vi "Zero Steer Jaguars.vi"() -> ()   [LabVIEW 2012]
uses:
  Controls/Zero Steer Jags Shifter.ctl
  <vilib>/Rock Robotics/SystemInterfaces/Utilities/FPGA_UtilitiesLED Source.ctl
  <vilib>/Rock Robotics/SystemInterfaces/Utilities/FPGA_UtilitiesLED State.ctl
  <vilib>/Rock Robotics/WPI/Joystick/WPI_JoystickGetSetRefNum.vi
  Globals/Potentiometers.vi
  Globals/Are We Calibrating Steering.vi
  Globals/Jaguar Commands.vi
  Globals/Motor Errors.vi
  Globals/Max Steer Voltage.vi
  <vilib>/Utility/file.llb/Write To Spreadsheet File (DBL).vi
  Globals/Pot Home Values.vi
panel:
  in  "Max Voltage":dbl
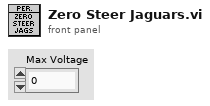
[diagram p1: front panel]
types:
  T1 = typedef "Zero Steer Jags Shifter.ctl" = enum16{"Wait for Button", "Move to Halfway", "Wait for Record"}
  T2 = typedef "WPI_JoystickDevRef.ctl" = cluster{"Device":T3}
  T3 = typedef "WPI_JoystickDeviceEnum.ctl" = enum16{"USB 1", "USB 2", "USB 3", "USB 4", "Kinect 1", "Kinect 2"}
  T4 = typedef "FPGA_UtilitiesLED State.ctl" = enum16{"Off", "On", "Toggle"}
  T5 = typedef "FPGA_UtilitiesLED Source.ctl" = enum16{"User LED", "FPGA LED"}
  T6 = typedef "WPI_AnalogChannelDevRef.ctl" = cluster{"DevStatus":errorcluster, "Analog Module":T7, "Analog Channel":T8}
  T7 = typedef "FPGA_TypedefAnalogModule.ctl" = enum16{"Analog Module 1", "Analog Module 2"}
  T8 = typedef "FPGA_AIChannel.ctl" = enum8{"AI 1", "AI 2", "AI 3", "AI 4", "AI 5", "AI 6", "AI 7", "AI 8", "Invalid"}
  T9 = cluster{"Front Left":T6, "Front Right":T6, "Rear Left":T6, "Rear Right":T6, "Actuator":T6}
  T10 = typedef "WPI_JoystickButtonState.ctl" = cluster{"Button 1":bool, "Button 2":bool, "Button 3":bool, "Button 4":bool, "Button 5":bool, "Button 6":bool, "Button 7":bool, "Button 8":bool, "Button 9":bool, "Button 10":bool, "Button 11":bool, "Button 12":bool}
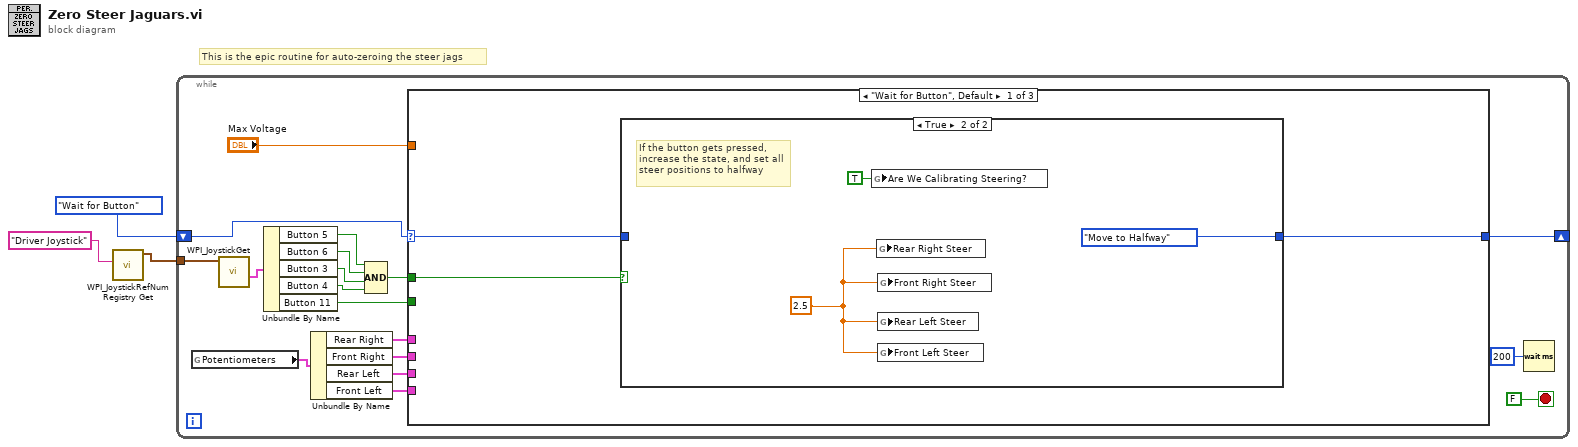
[diagram p0: block diagram]
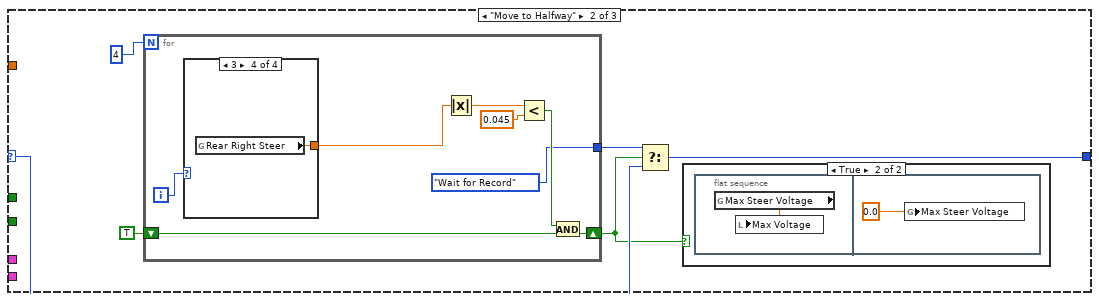
[diagram p3: hidden frame]
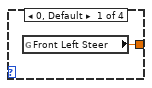
[diagram p5: hidden frame]
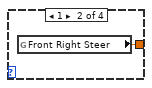
[diagram p6: hidden frame]
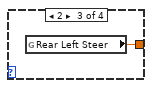
[diagram p7: hidden frame]
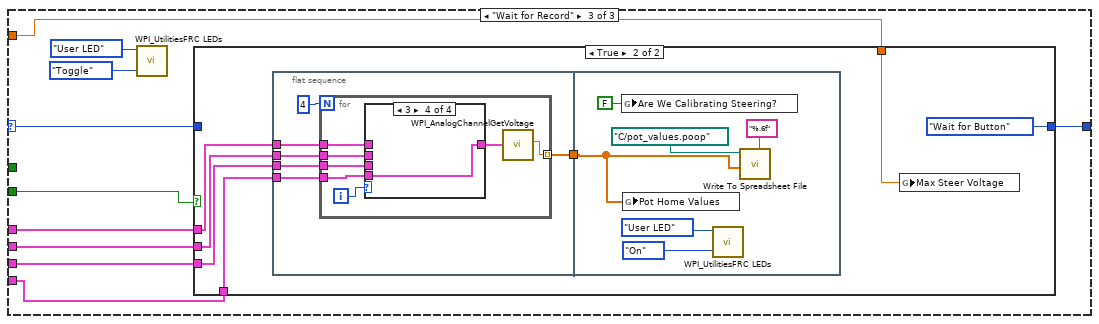
[diagram p8: hidden frame]
diagram:
  # "This is the epic routine for auto-zeroing the steer jags"
  n1 = call <vilib>:"WPI_JoystickRefNum Registry Get.vi"("refnum name"="Driver Joystick") -> ("JoystickDevRef"=w3:T2)  [unwired: 1 in, 9 out]
  n2 = while {
    tunnel: w3 -> [w15]
    shift-right: [w19] -> _
    shift-left: Zero_Steer_Jags_Shifter."Wait for Button" ("States") -> [w20]
    stop <- FALSE stop-if-true
    n3 = global read "Potentiometers.vi" "Potentiometers"() -> (w9:T9)
    n4 = call <vilib>:"WPI_JoystickGet.vi"("JoystickDevRef"=w15) -> ("Buttons"=w17:T10)  [unwired: 4 in, 2 out]
    n5 = Unbundle By Name(w17) -> ("Button 5"=w13:bool, "Button 6"=w12:bool, "Button 3"=w16:bool, "Button 4"=w11:bool, "Button 11"=w10:bool)
    n6 = Unbundle By Name(w9) -> ("Rear Right"=w8:T6, "Front Right"=w7:T6, "Rear Left"=w6:T6, "Front Left"=w5:T6)
    n7 = Compound Arithmetic op=AND(w13, w12, w16, w11) -> (w14:bool)
    n8 = case shown="\"Wait for Button\", Default" w20 {
      selector: w20 -> [w24 w31 w56]
      tunnel: [w23 w32 w55] -> w19
      tunnel: w14 -> [w22 _ _]
      tunnel: w10 -> [_ _ w54]
      tunnel: w8 -> [_ _ w53]
      tunnel: w7 -> [_ _ w52]
      tunnel: w6 -> [_ _ w51]
      tunnel: w5 -> [_ _ w50]
      tunnel: "Max Voltage" -> [_ _ w49]
      frame "Wait for Button", Default {
        n9 = case shown="True" w22 {
          tunnel: w24 -> [w25 _]
          tunnel: [w25 Zero_Steer_Jags_Shifter."Move to Halfway" ("States")] -> w23
          frame False {
          }
          frame True {
            w26 = 2.5 ("Front Right Steer")
            # "If the button gets pressed, \nincrease the state, and set all\nsteer positions to halfway"
            n10 = global write "Are We Calibrating Steering.vi" "Are We Calibrating Steering?"(TRUE ("Are We Calibrating Steering?")) -> ()
            n11 = global write "Jaguar Commands.vi" "Rear Right Steer"(w26) -> ()
            n12 = global write "Jaguar Commands.vi" "Front Right Steer"(w26) -> ()
            n13 = global write "Jaguar Commands.vi" "Rear Left Steer"(w26) -> ()
            n14 = global write "Jaguar Commands.vi" "Front Left Steer"(w26) -> ()
          }
        }
      }
      frame "Move to Halfway" {
        n15 = for {
          N: 4 -> [_]
          shift-right: [w42] -> w29
          shift-left: TRUE -> [w41]
          tunnel: [Zero_Steer_Jags_Shifter."Wait for Record" ("States")] -> w30
          i -> [w44]
          n16 = case shown="3" w44 {
            tunnel: [w45 w46 w47 w48] -> w37
            frame 0, Default {
              n17 = global read "Motor Errors.vi" "Front Left Steer"() -> (w45:dbl)
            }
            frame 1 {
              n18 = global read "Motor Errors.vi" "Front Right Steer"() -> (w46:dbl)
            }
            frame 2 {
              n19 = global read "Motor Errors.vi" "Rear Left Steer"() -> (w47:dbl)
            }
            frame 3 {
              n20 = global read "Motor Errors.vi" "Rear Right Steer"() -> (w48:dbl)
            }
          }
          n21 = Absolute Value(x=w37) -> (abs(x)=w38:dbl)
          n22 = Less?(x=w38, y=0.045) -> (x < y?=w40:bool)
          n23 = And(x=w40, y=w41) -> (x .and. y?=w42:bool)
        }
        n24 = Select(t=w30, s=w29, f=w31) -> (s? t:f=w32:T1)
        n25 = case shown="True" w29 {
          frame False {
          }
          frame True {
            n26 = flat-sequence {
              frame #0 {
                n27 = global read "Max Steer Voltage.vi" "Max Steer Voltage"() -> (w35:dbl)
                n28 = local write "Max Voltage"(w35) -> ()
              }
              frame #1 {
                n29 = global write "Max Steer Voltage.vi" "Max Steer Voltage"(0.0 ("Max Steer Voltage")) -> ()
              }
            }
          }
        }
      }
      frame "Wait for Record" {
        n30 = call <vilib>:"WPI_UtilitiesFRC LEDs.vi"("State"=FPGA_UtilitiesLED_State."Toggle", "LED Type"=FPGA_UtilitiesLED_Source."User LED") -> ()  [unwired: 8 in, 2 out]
        n31 = case shown="True" w54 {
          tunnel: w56 -> [w59 _]
          tunnel: [w59 Zero_Steer_Jags_Shifter."Wait for Button" ("States")] -> w55
          tunnel: w53 -> [_ w65]
          tunnel: w52 -> [_ w64]
          tunnel: w51 -> [_ w63]
          tunnel: w50 -> [_ w62]
          tunnel: w49 -> [_ w60]
          frame False {
          }
          frame True {
            n32 = flat-sequence {
              tunnel: w65 -> [w71]
              tunnel: w64 -> [w70]
              tunnel: w63 -> [w69]
              tunnel: w62 -> [w68]
              tunnel: [w67] -> w61
              tunnel: w61 -> [w84]
              frame #0 {
                n33 = for {
                  N: 4 -> [_]
                  tunnel: w71 -> [w78]
                  tunnel: w70 -> [w77]
                  tunnel: w69 -> [w76]
                  tunnel: w68 -> [w75]
                  tunnel: [w73] -> w67 mode=indexing
                  i -> [w79]
                  n34 = case shown="3" w79 {
                    tunnel: w78 -> [w80 _ _ _]
                    tunnel: w77 -> [_ w81 _ _]
                    tunnel: w76 -> [_ _ w82 _]
                    tunnel: w75 -> [_ _ _ w83]
                    tunnel: [w80 w81 w82 w83] -> w74
                    frame 0, Default {
                    }
                    frame 1 {
                    }
                    frame 2 {
                    }
                    frame 3 {
                    }
                  }
                  n35 = call <vilib>:"WPI_AnalogChannelGetVoltage.vi"("AIDeviceRef"=w74) -> ("Voltage"=w73:dbl)  [unwired: 8 in, 2 out]
                }
              }
              frame #1 {
                n36 = global write "Are We Calibrating Steering.vi" "Are We Calibrating Steering?"(FALSE ("Are We Calibrating Steering?")) -> ()
                n37 = global write "Pot Home Values.vi" "Pot Home Values"(w84) -> ()
                n38 = call <vilib>:"WPI_UtilitiesFRC LEDs.vi"("State"=FPGA_UtilitiesLED_State."On", "LED Type"=FPGA_UtilitiesLED_Source."User LED") -> ()  [unwired: 8 in, 2 out]
                n39 = call-poly <vilib>:"Write To Spreadsheet File.vi"("format (%.3f)"="%.6f", "1D data"=w84, "file path (dialog if empty)"=path "C:/pot_values.poop") -> ()  [unwired: 5 in, 1 out]
              }
            }
            n40 = global write "Max Steer Voltage.vi" "Max Steer Voltage"(w60) -> ()
          }
        }
      }
    }
    n41 = Wait (ms)(milliseconds to wait=u32 200) -> ()  [unwired: 1 out]
  }
